vi "Set Shooter Speed.vi"(11 "CAN Talon SRX Ref":T1) -> (3 "Flywheel RPM":dbl)   [LabVIEW 2016]
uses:
  <vilib>/Rock Robotics/WPI/MotorControl/WPI_MotorControlDeviceRef.ctl
  <vilib>/Rock Robotics/WPI/MotorControl/WPI_MotorControlType.ctl
  <vilib>/Rock Robotics/SystemInterfaces/DIO/FPGA_DIOPWMChannel.ctl
  <vilib>/Rock Robotics/WPI/PWM/WPI_PWMDeadband.ctl
  <vilib>/Rock Robotics/WPI/ThirdParty/CanMotor/TalonSRX/WPI_CANTalonSRX_APIControlMode.ctl
  Robot Global Data.vi
  <vilib>/Rock Robotics/Network Tables/NT Write Number.vi
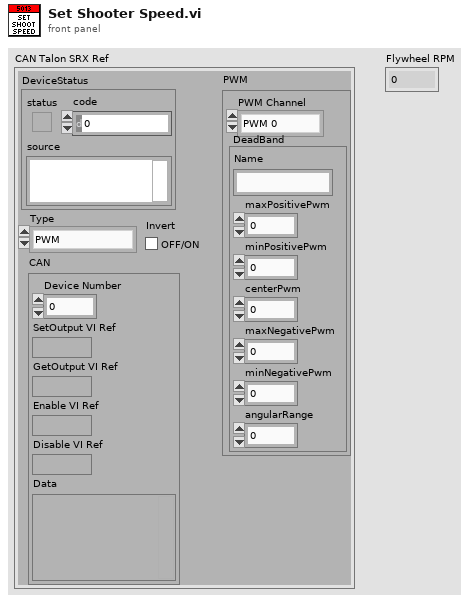
[diagram p1: front panel]
types:
  T1 = typedef "WPI_MotorControlDeviceRef.ctl" = cluster{"DeviceStatus":errorcluster, "Type":T2, "PWM":cluster{"PWM Channel":T3, "DeadBand":T4}, "CAN":cluster{"Device Number":u8, "SetOutput VI Ref":variant, "GetOutput VI Ref":variant, "Enable VI Ref":variant, "Disable VI Ref":variant, "Data":variant}, "Invert":bool}
  T2 = typedef "WPI_MotorControlType.ctl" = enum16{"PWM", "CAN"}
  T3 = typedef "FPGA_DIOPWMChannel.ctl" = enum8{"PWM 0", "PWM 1", "PWM 2", "PWM 3", "PWM 4", "PWM 5", "PWM 6", "PWM 7", "PWM 8", "PWM 9", "PWM MXP 0", "PWM MXP 1", "PWM MXP 2", "PWM MXP 3", "PWM MXP 4", "PWM MXP 5", "PWM MXP 6", "PWM MXP 7", "PWM MXP 8", "PWM MXP 9", "Invalid"}
  T4 = typedef "WPI_PWMDeadband.ctl" = cluster{"Name":string, "maxPositivePwm":i32, "minPositivePwm":i32, "centerPwm":i32, "maxNegativePwm":i32, "minNegativePwm":i32, "angularRange":u16}
  T5 = typedef "WPI_CANTalonSRX_APIControlMode.ctl" = enum8{"Percent VBus", "Speed", "Position", "Slave", "Unchanged / Invalid", "Voltage Compensation", "Current", "Motion Profile", "Motion Magic"}
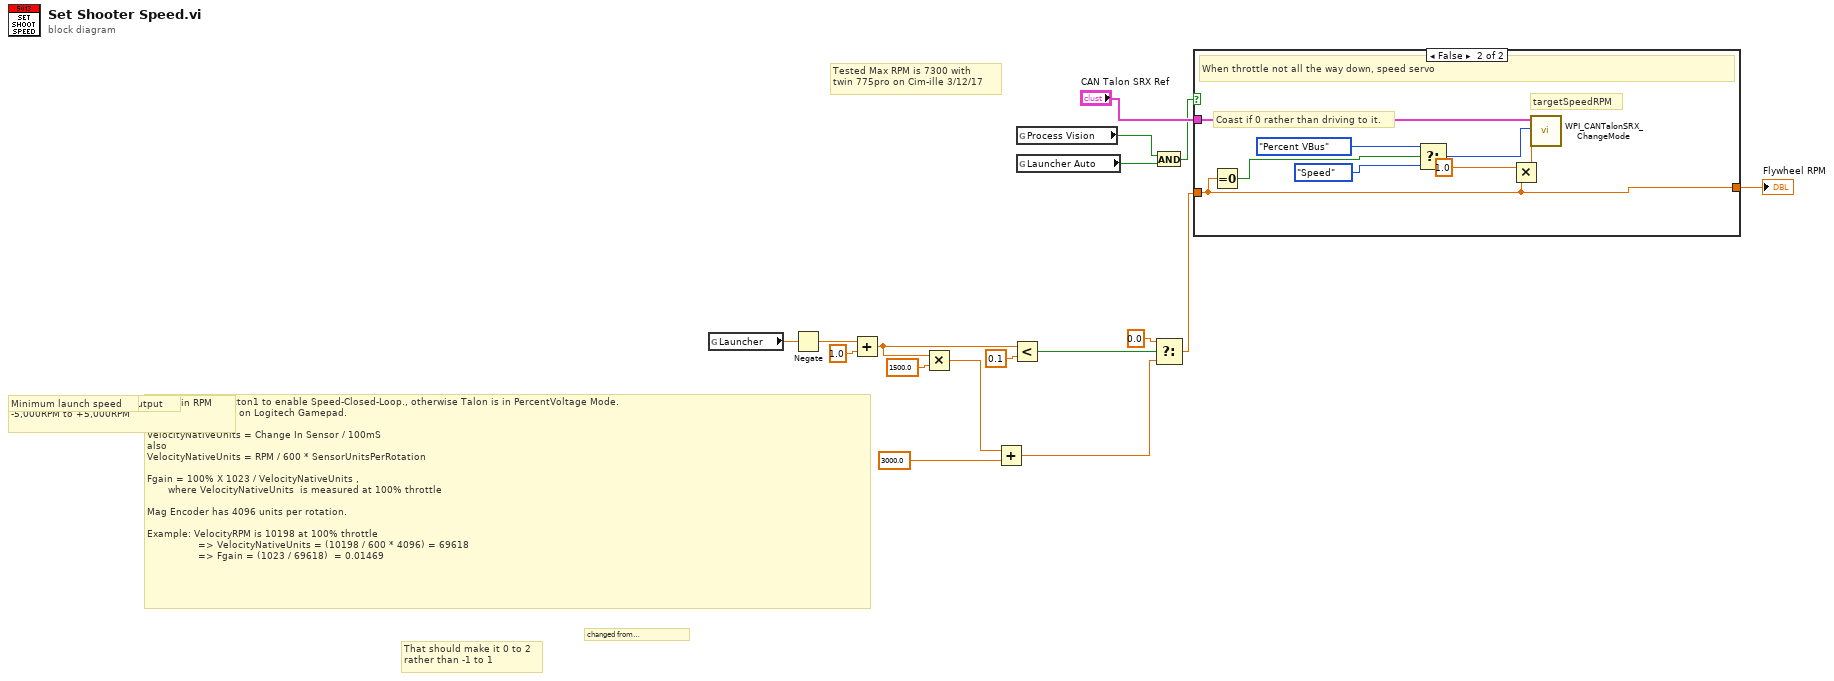
[diagram p0: block diagram]
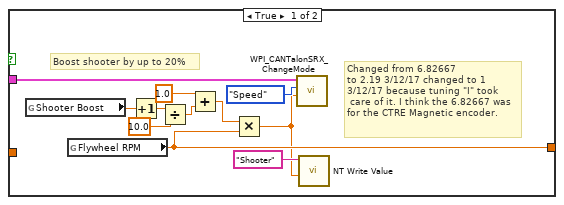
[diagram p2: hidden frame]
diagram:
  # "Tested Max RPM is 7300 with \ntwin 775pro on Cim-ille 3/12/17"
  # "changed from\n0 to 2500 on 3/3/17"
  # "Minimum launch speed"
  # "That should make it 0 to 2\nrather than -1 to 1"
  # "Press and Hold Button1 to enable Speed-Closed-Loop., otherwise Talon is in PercentVoltage Mode.  \nUse the Left Y-axis on Logitech Gamepad.\n\nVelocityNativeUnits = Change In Sensor / 100mS\nalso\nVelocityNativeUnits = RPM / 600 * SensorUnitsPerRotation\n\nFgain = 100% X 1023 / VelocityNativeUnits , \n       where VelocityNativeUnits  is measured at 100% throttle\n\nMag Encoder has 4096 units per rotation.\n\nExample: VelocityRPM is 10198 at 100% throttle\n                 => VelocityNativeUnits = (10198 / 600 * 4096) = 69618\n                 => Fgain = (1023 / 69618)  = 0.01469"
  # "Joystick directly controls output"
  # "Calculate what Velocity to servo to in RPM\n-5,000RPM to +5,000RPM"
  n1 = global read "Robot Global Data.vi" "Launcher"() -> (w6:dbl)
  n2 = Negate(x=w6) -> (-x=w5:dbl)
  n3 = Add(x=w5, y=1.0) -> (x+y=w11:dbl)
  n4 = Multiply(x=w11, y=1500.0) -> (x*y=w16:dbl)
  n5 = Add(x=w16, y=3000.0) -> (x+y=w4:dbl)
  n6 = Less?(x=w11, y=0.1) -> (x < y?=w8:bool)
  n7 = global read "Robot Global Data.vi" "Process Vision"() -> (w2:bool)
  n8 = global read "Robot Global Data.vi" "Launcher Auto"() -> (w1:bool)
  n9 = And(x=w2, y=w1) -> (x .and. y?=w3:bool)
  n10 = Select(t=0.0, s=w8, f=w4) -> (s? t:f=w9:dbl)
  n11 = case shown="False" w3 {
    tunnel: w9 -> [_ w31]
    tunnel: "CAN Talon SRX Ref" -> [w26 w36]
    tunnel: [w27 w31] -> w17
    frame True {
      # "Boost shooter by up to 20%"
      # "Changed from 6.82667\nto 2.19 3/12/17 changed to 1\n3/12/17 because tuning \"I\" took\n care of it. I think the 6.82667 was\nfor the CTRE Magnetic encoder."
      n12 = global read "Robot Global Data.vi" "Shooter Boost"() -> (w25:dbl)
      n13 = global read "Robot Global Data.vi" "Flywheel RPM"() -> (w27:dbl)
      n14 = Increment(x=w25) -> (x+1=w23:dbl)
      n15 = Divide(x=w23, y=10.0) -> (x/y=w21:dbl)
      n16 = Add(x=1.0, y=w21) -> (x+y=w20:dbl)
      n17 = Multiply(x=w20, y=w27) -> (x*y=w18:dbl)
      n18 = call <vilib>:"WPI_CANTalonSRX_ChangeMode.vi"("Output"=w18, "Control Mode"=WPI_CANTalonSRX_APIControlMode."Speed", "CAN Talon SRX Ref"=w26) -> ()  [unwired: 7 in, 2 out]
      n19 = call-poly <vilib>:"NT Write Value.vi"("Numeric"=w18, "Name"="Shooter") -> ()  [unwired: 9 in, 1 out]
    }
    frame False {
      # "Coast if 0 rather than driving to it."
      # "targetSpeedRPM"
      # "When throttle not all the way down, speed servo"
      n20 = Equal To 0?(x=w31) -> (x = 0?=w32:bool)
      n21 = Select(t=WPI_CANTalonSRX_APIControlMode."Percent VBus" ("Control Mode"), s=w32, f=WPI_CANTalonSRX_APIControlMode."Speed" ("Control Mode")) -> (s? t:f=w35:T5)
      n22 = Multiply(x=1.0, y=w31) -> (x*y=w30:dbl)
      n23 = call <vilib>:"WPI_CANTalonSRX_ChangeMode.vi"("Output"=w30, "Control Mode"=w35, "CAN Talon SRX Ref"=w36) -> ()  [unwired: 7 in, 2 out]
    }
  }
  "Flywheel RPM" <- w17
